vi "Switch On Off.vi"(8 "error in (no error)":errorcluster, 10 "Switch Mode":bool=TRUE caption="Switch On ? (T: Yes)", 11 "VISA resource name":refnum<visa-resource-name>) -> (0 "error out":errorcluster, 3 "VISA resource name out":refnum<visa-resource-name>)   [LabVIEW 2014, in "Fluke 190 Series II.lvlib"]
doc: "Switches the Scopemeter on or off."
uses:
  Fluke 190 Series II.lvlib
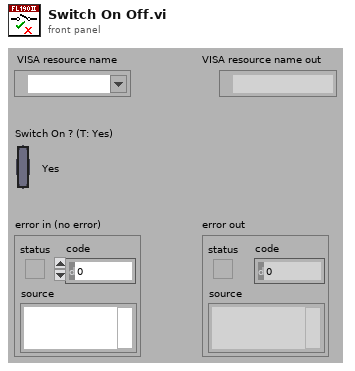
[diagram p1: front panel]
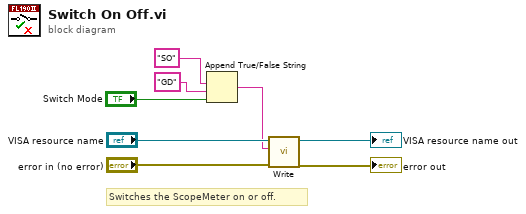
[diagram p0: block diagram]
diagram:
  # "Switches the ScopeMeter on or off."
  n1 = Append True/False String(1:"Switch Mode", 2:"GD", 3:"SO") -> (0:w1:string)  [unwired: 1 in]
  n2 = call "Write.vi"("error in (no error)"="error in (no error)", "Write Buffer"=w1, "VISA resource name"="VISA resource name") -> ("error out"=→"error out":errorcluster, "VISA resource name out"=→"VISA resource name out":refnum<visa-resource-name>)  [unwired: 7 out]
